vi "Monitor Test.vi"() -> ()   [LabVIEW 2017]
uses:
  <vilib>/Utility/miscctls.llb/LVAllMonitorsDisplayTypeDef.ctl
  System.Windows.Forms
  System.Drawing
panel:
  out "Monitor H and W":i32[][](array[numeric])
  out "Display Names":string[](array[string])
  out "# of Attached Monitor":i32
  out "Primary Monitor\nMethod 1":i32
  out "Monitors Info []":T1
  out "Primary Monitor\nMethod 2":i32
  out "Current Monitor":u16
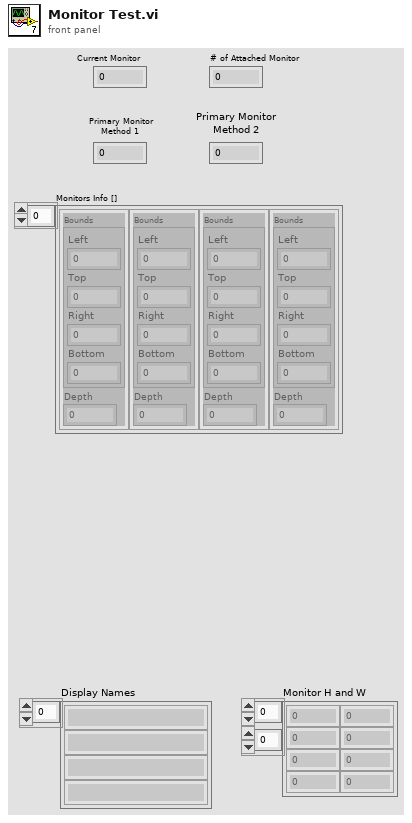
[diagram p1: front panel]
types:
  T1 = typedef "LVAllMonitorsDisplayTypeDef.ctl" = cluster{"Bounds":cluster{"Left":i16, "Top":i16, "Right":i16, "Bottom":i16}, "Depth":i16}[]
  T2 = typedef "LVRectTypeDef.ctl" = cluster{"Left":i16, "Top":i16, "Right":i16, "Bottom":i16}
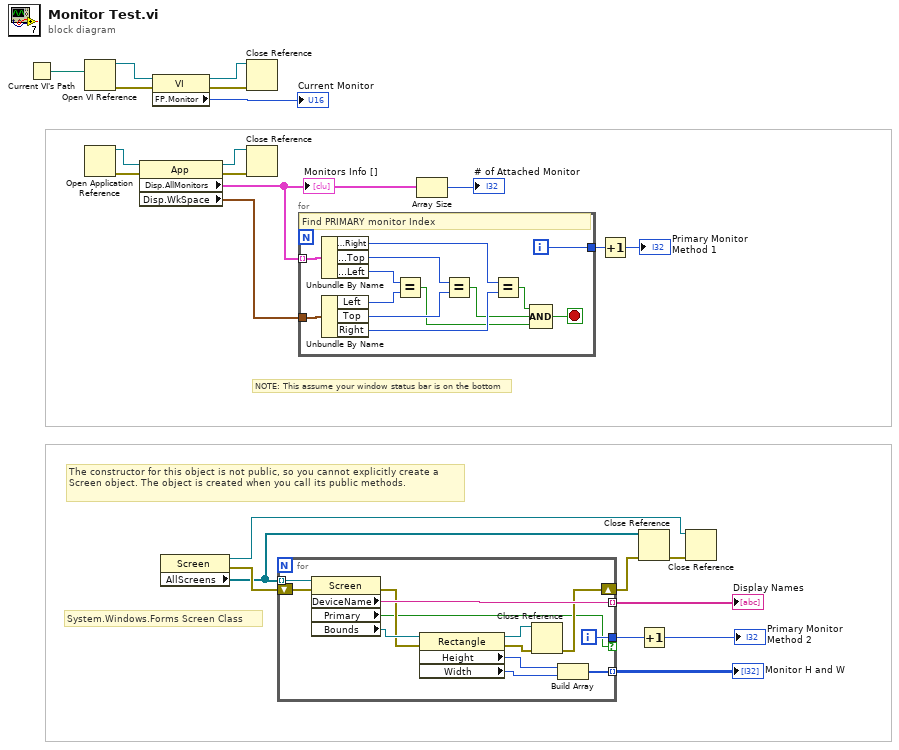
[diagram p0: block diagram]
diagram:
  # "NOTE: This assume your window status bar is on the bottom"
  # "System.Windows.Forms Screen Class"
  # "The constructor for this object is not public, so you cannot explicitly create a Screen object. The object is created when you call its public methods."
  n1 = Current VI's Path() -> (path=w19:path)
  n2 = Open VI Reference(vi path=w19) -> (vi reference=w24:refnum<vi>, error out=w23:errorcluster)  [unwired: 5 in]
  n3 = Open Application Reference() -> (0:w17:errorcluster, 3:w16:refnum<vi>)  [unwired: 4 in]
  n4 = property class="App"(reference=w16, error in=w17) -> (reference out=w10:refnum<vi>, error out=w18:errorcluster, "Disp.AllMonitors"=w11:T1, "Disp.WkSpace"=w15:T2)
  "Monitors Info []" <- w11
  n5 = property class="VI"(reference=w24, error in=w23) -> (reference out=w21:refnum<vi>, error out=w22:errorcluster, "FP.Monitor"=→"Current Monitor":u16)
  n6 = property class="Screen"() -> (reference out=w4:refnum<k24>, error out=w8:errorcluster, "AllScreens"=w6:refnum<k24>[])  [unwired: 2 in]
  n7 = Close Reference(reference=w21, error in (no error)=w22) -> ()  [unwired: 1 out]
  n8 = Close Reference(reference=w10, error in (no error)=w18) -> ()  [unwired: 1 out]
  n9 = for {
    tunnel: w6 -> [w37] mode=indexing
    tunnel: [w36] -> w9 mode=indexing
    shift-right: [w30] -> w7
    shift-left: w8 -> [w34]
    tunnel: [w29] -> w3 if=w28
    tunnel: [w25] -> w2 mode=indexing
    i -> [w29]
    n10 = property class="Screen"(reference=w37, error in=w34) -> (error out=w31:errorcluster, "DeviceName"=w36:string, "Primary"=w28:bool, "Bounds"=w35:refnum<k24>)  [unwired: 1 out]
    n11 = property class="Rectangle"(reference=w35, error in=w31) -> (reference out=w32:refnum<k24>, error out=w33:errorcluster, "Height"=w27:i32, "Width"=w26:i32)
    n12 = Close Reference(reference=w32, error in (no error)=w33) -> (error out=w30:errorcluster)
    n13 = Build Array(w27, w26) -> (w25:i32[])
  }
  "Display Names" <- w9
  "Monitor H and W" <- w2
  n14 = for {
    tunnel: w11 -> [w50] mode=indexing
    tunnel: w15 -> [w49]
    tunnel: [w39] -> w14
    i -> [w39]
    stop <- w38 stop-if-true
    # "Find PRIMARY monitor Index"
    n15 = Unbundle By Name(w50) -> ("Bounds.Right"=w44:i16, "Bounds.Top"=w46:i16, "Bounds.Left"=w48:i16)
    n16 = Unbundle By Name(w49) -> ("Left"=w47:i16, "Top"=w45:i16, "Right"=w43:i16)
    n17 = Equal?(x=w48, y=w47) -> (x = y?=w40:bool)
    n18 = Equal?(x=w46, y=w45) -> (x = y?=w41:bool)
    n19 = Equal?(x=w44, y=w43) -> (x = y?=w42:bool)
    n20 = Compound Arithmetic op=AND(w42, w41, w40) -> (w38:bool)
  }
  n21 = Array Size(array=w11) -> (size(s)=→"# of Attached Monitor":i32)
  n22 = Increment(x=w14) -> (x+1=→"Primary Monitor\nMethod 1":i32)
  n23 = Close Reference(reference=w6, error in (no error)=w7) -> (error out=w5:errorcluster)
  n24 = Increment(x=w3) -> (x+1=→"Primary Monitor\nMethod 2":i32)
  n25 = Close Reference(reference=w4, error in (no error)=w5) -> ()  [unwired: 1 out]
